vi "Send Class Loading Result.vi"(5 "Class Names":string[](array[string]), 7 "Priority":T2=enum."Normal" caption="Message Priority (Normal)", 8 "error in (no error)":errorcluster, 9 "Class Array":refnum<class>[](array[class]), 10 "Classes Map":T1, 11 "Message Enqueuer in":refnum<class "Message Enqueuer.lvclass">) -> (0 "error out":errorcluster, 3 "Message Enqueuer out":refnum<class "Message Enqueuer.lvclass">)   [LabVIEW 2023, in "Class Loader Interfaces.lvlib" / "Class Loading Result Msg.lvclass"]
doc: "Sends the <b>Class Loader Interfaces.lvlib:Class Loading Result Msg.lvclass</b> message.\n\nThis message will call <b>Class Loading Result.vi</b> on the <b>Class Loader Interfaces.lvlib:Class Loader Interfaces.lvclass</b> actor.\n\n<b>Class Loading Result.vi Description</b>"
uses:
  Class Loading Result Msg.lvclass
  Class Loading Result Msg.lvclass/Class Loading Result Msg.ctl
  <vilib>/ActorFramework/Message Enqueuer/Message Enqueuer.lvclass
  C:/Program Files/National Instruments/LabVIEW 2023/vi.lib/ActorFramework/Message/Message.lvclass
  C:/Projects/Shared Libraries/Class Loader/Class Loader/Class Loader Interfaces/Class Loader Interfaces Messages/Class Loading Result Msg/Class Loading Result Msg.lvclass
  <vilib>/ActorFramework/Message Enqueuer/Message Priority.ctl
  Class Loader/Classes Map.ctl
  Class Loader/Class Loader.lvclass
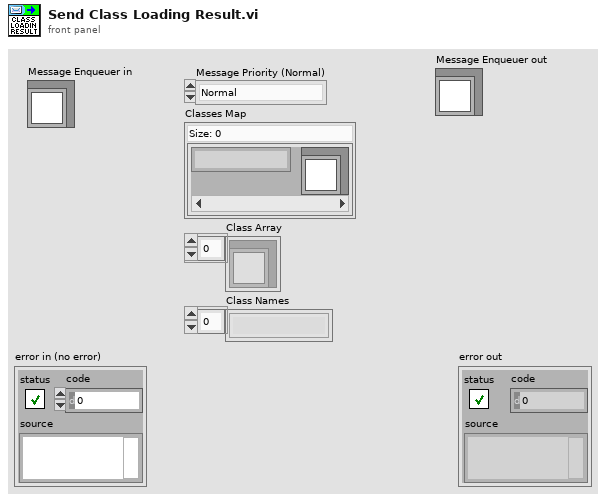
[diagram p1: front panel]
types:
  T1 = typedef "Class Loader.lvlib/Class Loader.lvclass/Classes Map.ctl" = map{string, refnum<class>}
  T2 = typedef "Actor Framework.lvlib/Message Enqueuer.lvclass/Message Priority.ctl" = enum16{"Low", "Normal", "High"}
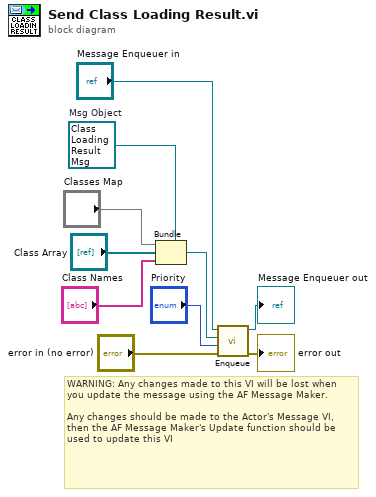
[diagram p0: block diagram]
diagram:
  w7 = refnum<class "Class Loading Result Msg.lvclass"> refnum  # Msg Object
  # "WARNING: Any changes made to this VI will be lost when you update the message using the AF Message Maker.\n\nAny changes should be made to the Actor's Message VI, then the AF Message Maker's Update function should be used to update this VI"
  n1 = Bundle(cluster=w7, "Classes Map", "Class Array", "Class Names") -> (w2:refnum<class "Class Loading Result Msg.lvclass">)
  n2 = call <vilib>:"Enqueue.vi"("error in (no error)"="error in (no error)", "Message Priority (Normal)"="Priority", "Message"=w2, "Message Enqueuer in"="Message Enqueuer in") -> ("error out"=→"error out":errorcluster, "Message Enqueuer out"=→"Message Enqueuer out":refnum<class "Message Enqueuer.lvclass">)  [unwired: 6 in]
